vi "Clear Table.vi"(1 "Data IN":T1 caption="Data") -> (0 "Data OUT":T1 caption="Data")   [LabVIEW 2012]
uses:
  PDF Table Data.ctl
  C:/Users/MaxCorp/Documents/TopPerm - Base/DLL/itextsharp.dll
  DLL/itextsharp.dll
  PDF Table XControl.xctl
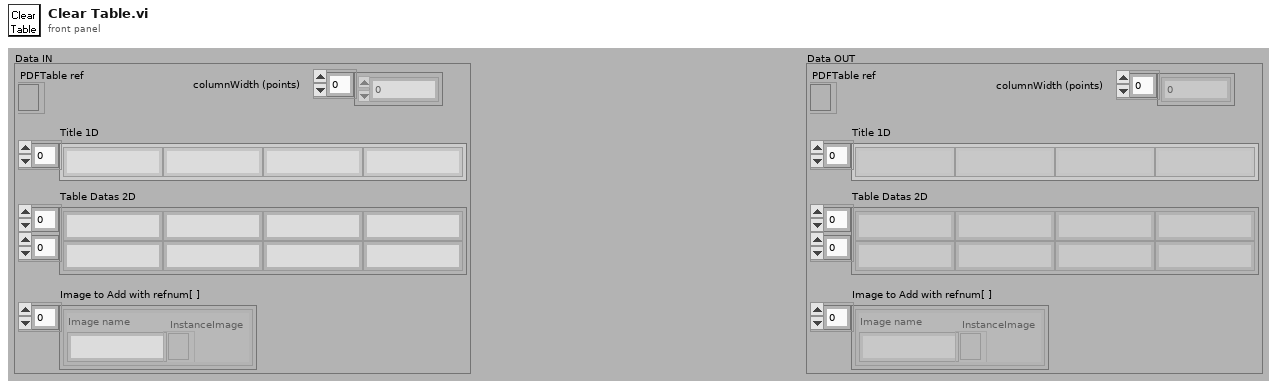
[diagram p1: front panel]
types:
  T1 = typedef "PDF Table XControl.xctl/PDF Table Data.ctl" = cluster{"PDFTable ref":refnum<k24>, "columnWidth (points)":sgl[], "Title 1D":string[], "Table Datas 2D":string[][], "Image to Add with refnum[ ]":cluster{"Image name":string, "InstanceImage":refnum<k24>}[]}
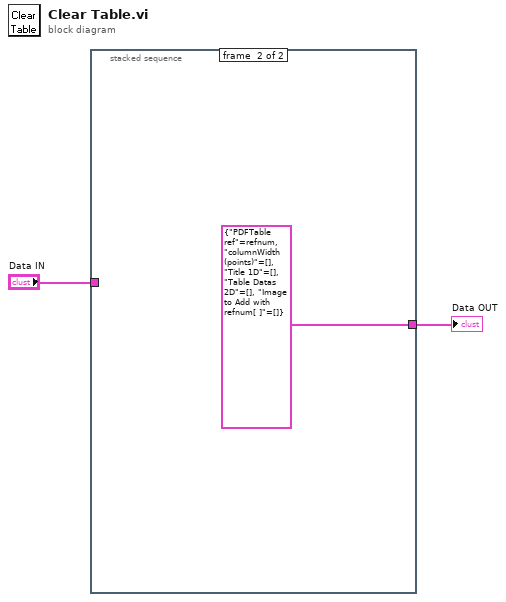
[diagram p0: block diagram]
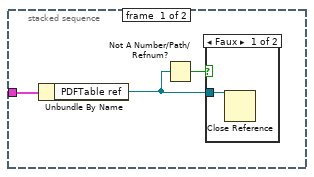
[diagram p2: hidden frame]
diagram:
  n1 = stacked-sequence {
    tunnel: "Data IN" -> [w5 _]
    tunnel: [_ T1 {"PDFTable ref"=refnum, "columnWidth (points)"=[], "Title 1D"=[], "Table Datas 2D"=[], "Image to Add with refnum[ ]"=[]} ("Data OUT")] -> w1
    frame #0 {
      n2 = Unbundle By Name(w5) -> ("PDFTable ref"=w3:refnum<k24>)
      n3 = Not A Number/Path/Refnum?(number/path/refnum=w3) -> (NaN/Path/Refnum?=w4:bool)
      n4 = case shown="Faux" w4 {
        tunnel: w3 -> [w6 _]
        frame False {
          n5 = Close Reference(reference=w6) -> ()  [unwired: 1 in, 1 out]
        }
        frame True {
        }
      }
    }
    frame #1 {
    }
  }
  "Data OUT" <- w1
